vi "Strain - Continuous Input.vi"() -> ()   [LabVIEW 2022 SP3]
doc: "This example demonstrates how to continuously acquire buffered strain measurements using a DAQmx device.\n\nFor instructions on how to connect your signals to the DAQ device, refer to your device documentation."
uses:
  <vilib>/Utility/error.llb/DialogType.ctl
  <vilib>/DAQmx/read.llb/DAQmx Read (Analog 1D Wfm NChan NSamp).vi
  <vilib>/DAQmx/create/channels.llb/DAQmx Create Channel (AI-Strain-Strain Gage).vi
  <vilib>/DAQmx/configure/timing.llb/DAQmx Timing (Sample Clock).vi
  <vilib>/DAQmx/configure/task.llb/DAQmx Configure Logging (TDMS).vi
  <vilib>/DAQmx/configure/trigger.llb/DAQmx Start Trigger (Digital Edge).vi
  <vilib>/DAQmx/configure/trigger.llb/DAQmx Start Trigger (Time).vi
  <vilib>/DAQmx/configure/trigger.llb/DAQmx Start Trigger (Analog Edge).vi
  <vilib>/DAQmx/calibration/calibrationInfo.llb/DAQmx Perform Shunt Calibration Ex (Strain).vi
  <vilib>/DAQmx/miscellaneous.llb/DAQmx Fill In Error Info.vi
  <resource>/objmgr/daqmx.rc
panel:
  in  "Trigger Type":T1(tab)
  in  "Digital Start Trigger Edge":i32(ring)=10280 caption="Edge" items=["Rising"=10280, "Falling"=10171]
  in  "Digital Start Trigger Source":tag="/Dev1/PFI0" caption="Source"
  in  "Digital Pause Trigger Pause When":i32(ring)=10192 caption="Pause When" items=["High"=10192, "Low"=10214]
  in  "Digital Pause Trigger Source":tag="/Dev1/PFI0" caption="Source"
  in  "Analog Start Trigger Level":dbl caption="Level" format="%0.2f"
  in  "Analog Start Trigger Hysteresis":dbl caption="Hysteresis" format="%.2f"
  in  "Analog Start Trigger Slope":i32(ring)=10280 caption="Slope" items=["Rising"=10280, "Falling"=10171]
  in  "Analog Start Trigger Source":string="APFI0" caption="Source"
  in  "Analog Pause Trigger Source":string="APFI0" caption="Source"
  in  "Analog Pause Trigger Pause When":i32(ring)=10093 caption="Pause When" items=["Above Level"=10093, "Below Level"=10107]
  in  "Analog Pause Trigger Level":dbl caption="Level" format="%.2f"
  in  "When":timestamp
  in  "Select Time\nManually":bool
  in  "Strain Gage Information":T2={"Gage Factor"=2.0, "Nominal Gage Resistance"=350.0, "Poisson Ratio"=0.3} {"Nominal Gage Resistance" format="%0.2f"; "Poisson Ratio" format="%0.2f"; "Gage Factor" format="%0.2f"}
  in  "Bridge Information":T3={"Strain Configuration"=10183, "Lead Wire Resistance"=0.0, "Initial Bridge Voltage"=0.0, "Voltage Excitation Source"=10200, "Voltage Excitation Value"=2.5} {"Initial Bridge Voltage" format="%0.2f"; "Voltage Excitation Source" items=["Internal"=10200, "External"=10167, "None"=10230]; "Voltage Excitation Value" format="%0.2f"; "Lead Wire Resistance" format="%0.2f"; "Strain Configuration" items=["Full Bridge I"=10183, "Full Bridge II"=10184, "Full Bridge III"=10185, "Half Bridge I"=10188, "Half Bridge II"=10189, "Quarter Bridge I"=10271, "Quarter Bridge II"=10272]}
  in  "TDMS File Path":path
  in  "Logging Mode":i32(ring)=10231 items=["Off"=10231, "Log and Read"=15842]
  in  "Sample Clock Source":tag="OnboardClock"
  in  "Do Shunt Cal?":bool caption="Enable Shunt Cal"
  in  "Shunt Element Location":i32(ring)=12465 caption="shunt element location" items=["R1"=12465, "R2"=12466, "R3"=12467, "R4"=14813, "None"=10230]
  in  "Shunt Resistance":dbl=100000.0 format="%#.3p"
  in  "Do Offset Null?":bool caption="Enable Offset Null"
  in  "Minimum Value":dbl=-0.001
  in  "Maximum Value":dbl=0.001
  in  "Physical Channel":tag="Dev1/ai0"
  in  "Stop":bool
  out "Waveform Chart":waveform(dbl)[](graph)
  in  "Samples per Loop":i32=100
  in  "Sample Rate":dbl=1000.0
  out "Actual Sample Rate":dbl format="%0.2f"
  # "Channel Settings"
  # "Acquired Data"
  # "Trigger Settings"
  # "Shunt Calibration \nand Offset Null Settings"
  # "Timing Settings"
  # "Logging Settings"
  # "To enable triggers, select a tab above, and configure the settings.\n\nNot all hardware supports all trigger types. Refer to your device documentation for more information."
  # "This trigger type is not supported in continuous sample timing. \n\nRefer to your device documentation for more information on which triggers are supported."
  # "This trigger type is not supported in continuous sample timing. \n\nRefer to your device documentation for more information on which triggers are supported."
  # "If time is not manually set, task will begin after 10 seconds"
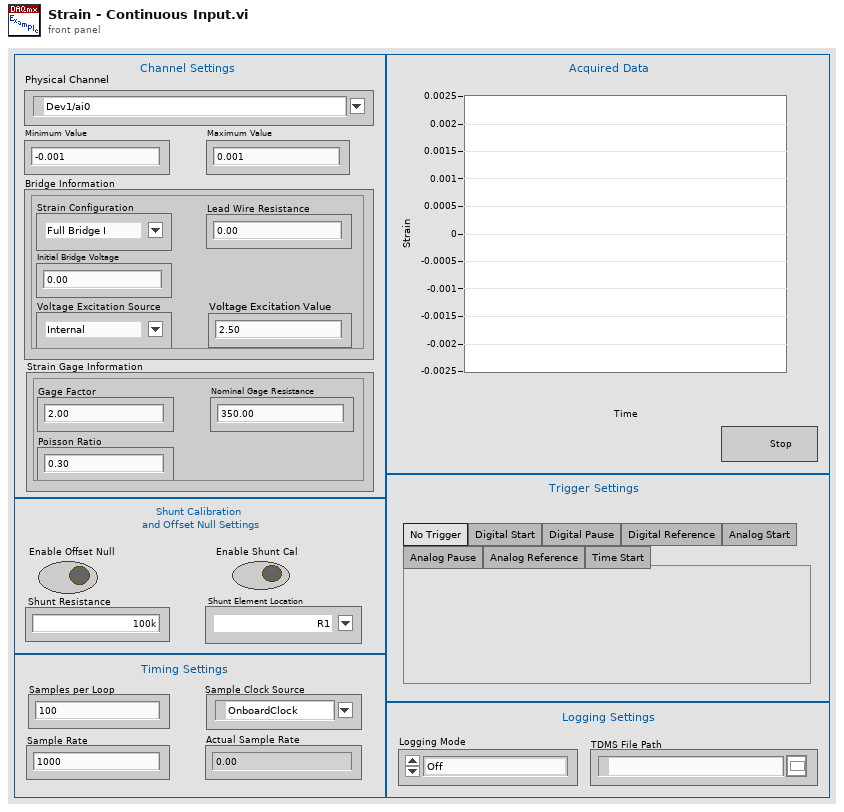
[diagram p1: front panel]
types:
  T1 = enum32{"No Trigger", "Digital Start", "Digital Pause", "Digital Reference", "Analog Start", "Analog Pause", "Analog Reference", "Time Start"}
  T2 = cluster{"Gage Factor":dbl, "Nominal Gage Resistance":dbl, "Poisson Ratio":dbl}
  T3 = cluster{"Strain Configuration":i32, "Lead Wire Resistance":dbl, "Initial Bridge Voltage":dbl, "Voltage Excitation Source":i32, "Voltage Excitation Value":dbl}
  T4 = typedef "DialogType.ctl" = u16
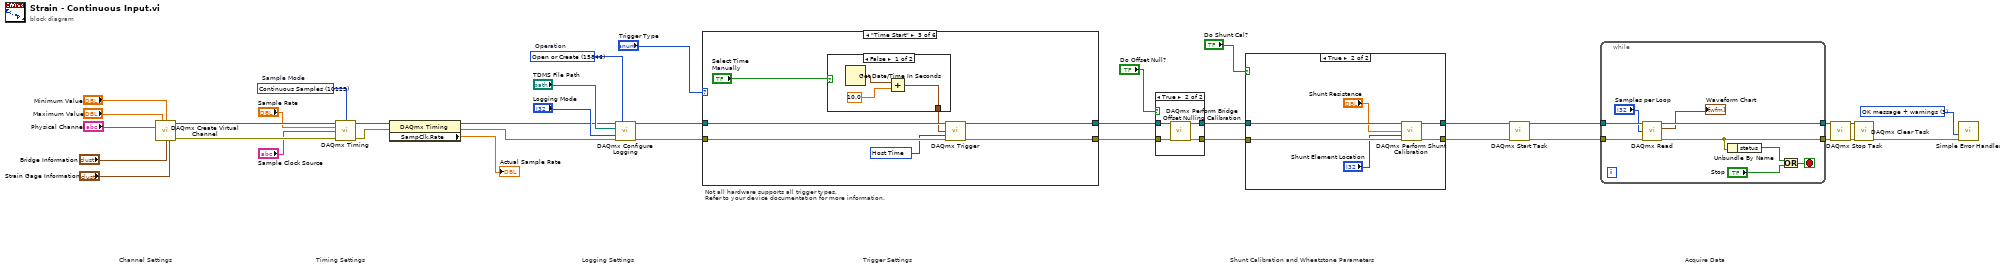
[diagram p0: block diagram]
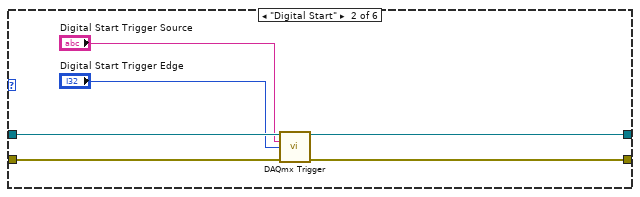
[diagram p3: hidden frame]
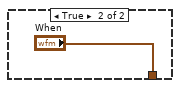
[diagram p4: hidden frame]
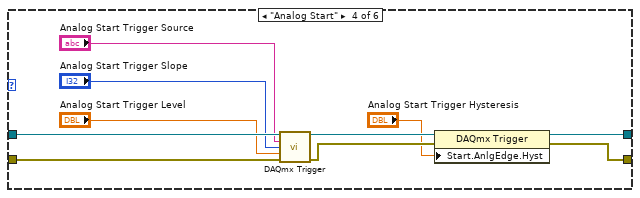
[diagram p5: hidden frame]
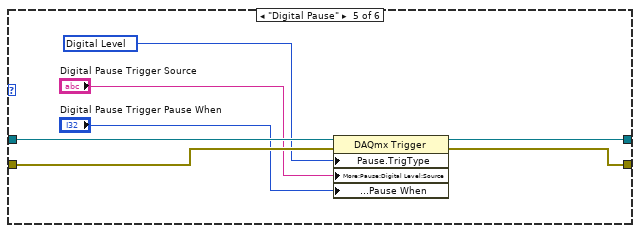
[diagram p6: hidden frame]
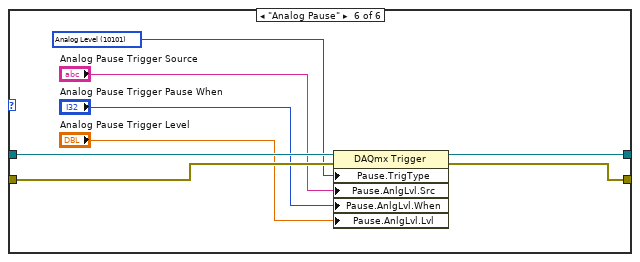
[diagram p7: hidden frame]
diagram:
  w6 = T4 3 items=["no dialog", "OK message", "continue or stop message", "OK message + warnings", "continue/stop + warnings"] ("type of dialog (OK msg:1)")
  w15 = 15846 items=["Open"=10437, "Open or Create"=15846, "Create or Replace"=15847, "Create"=15848]  # Operation
  w35 = 10123 items=["Finite Samples"=10178, "Continuous Samples"=10123, "Hardware Timed Single Point"=12522]  # Sample Mode
  # "Trigger Settings"
  # "Not all hardware supports all trigger types.\nRefer to your device documentation for more information."
  # "Logging Settings"
  # "Acquire Data"
  # "Shunt Calibration and Wheatstone Parameters"
  # "Timing Settings"
  # "Channel Settings"
  n1 = call-poly <vilib>:"DAQmx Create Virtual Channel.vi"("maximum value"="Maximum Value", "minimum value"="Minimum Value", "physical channels"="Physical Channel", "bridge information"="Bridge Information", "strain gage information"="Strain Gage Information") -> ("task out"=w33:refnum<k21>, "error out"=w34:errorcluster)  [unwired: 9 in]
  n2 = call-poly <vilib>:"DAQmx Timing.vi"("task/channels in"=w33, "sample mode"=w35, "rate"="Sample Rate", "source"="Sample Clock Source", "error in"=w34) -> ("task out"=w37:refnum<k21>, "error out"=w36:errorcluster)  [unwired: 9 in]
  n3 = property class="DAQmx Timing"(reference=w37, error in=w36) -> (reference out=w14:refnum<k21>, error out=w13:errorcluster, "SampClk.Rate"=→"Actual Sample Rate":dbl)
  n4 = call-poly <vilib>:"DAQmx Configure Logging.vi"("task/channels in"=w14, "operation"=w15, "file path"="TDMS File Path", "logging mode"="Logging Mode", "error in"=w13) -> ("task out"=w3:refnum<k21>, "error out"=w4:errorcluster)  [unwired: 9 in]
  n5 = case shown="\"Time Start\"" "Trigger Type" {
    tunnel: w3 -> [w39 w45 w52 w66 w73 w81]
    tunnel: w4 -> [w38 w44 w51 w65 w70 w78]
    tunnel: [w39 w43 w50 w63 w72 w80] -> w2
    tunnel: [w38 w42 w49 w62 w71 w79] -> w1
    frame "No Trigger", Default {
    }
    frame "Digital Start" {
      n6 = call-poly <vilib>:"DAQmx Trigger.vi"("task/channels in"=w45, "source"="Digital Start Trigger Source", "edge"="Digital Start Trigger Edge", "error in"=w44) -> ("task out"=w43:refnum<k21>, "error out"=w42:errorcluster)  [unwired: 10 in]
    }
    frame "Time Start" {
      w48 = 16126 items=["Host Time"=16126, "I/O Device Time"=16127] ("timescale")
      n7 = case shown="False" "Select Time\nManually" {
        tunnel: [w54 "When"] -> w46
        frame False {
          n8 = Get Date/Time In Seconds() -> (seconds since 1Jan1904=w55:timestamp)
          n9 = Add(x=w55, y=10.0) -> (x+y=w54:timestamp)
        }
        frame True {
        }
      }
      n10 = call-poly <vilib>:"DAQmx Trigger.vi"("task/channels in"=w52, "when"=w46, "timescale"=w48, "error in"=w51) -> ("task out"=w50:refnum<k21>, "error out"=w49:errorcluster)  [unwired: 10 in]
    }
    frame "Analog Start" {
      n11 = call-poly <vilib>:"DAQmx Trigger.vi"("task/channels in"=w66, "source"="Analog Start Trigger Source", "slope"="Analog Start Trigger Slope", "level"="Analog Start Trigger Level", "error in"=w65) -> ("task out"=w61:refnum<k21>, "error out"=w60:errorcluster)  [unwired: 9 in]
      n12 = property class="DAQmx Trigger"(reference=w61, error in=w60, "Start.AnlgEdge.Hyst"="Analog Start Trigger Hysteresis") -> (reference out=w63:refnum<k21>, error out=w62:errorcluster)
    }
    frame "Digital Pause" {
      w69 = 10152 items=["Analog Level"=10101, "Analog Window"=10103, "Digital Level"=10152, "Digital Pattern"=10398, "None"=10230] ("Pause.TrigType")
      n13 = property class="DAQmx Trigger"(reference=w73, error in=w70, "Pause.TrigType"=w69, "More:Pause:Digital Level:Source"="Digital Pause Trigger Source", "More:Pause:Digital Level:Pause When"="Digital Pause Trigger Pause When") -> (reference out=w72:refnum<k21>, error out=w71:errorcluster)
    }
    frame "Analog Pause" {
      w77 = 10101 items=["Analog Level"=10101, "Analog Window"=10103, "Digital Level"=10152, "Digital Pattern"=10398, "None"=10230] ("Pause.TrigType")
      n14 = property class="DAQmx Trigger"(reference=w81, error in=w78, "Pause.TrigType"=w77, "Pause.AnlgLvl.Src"="Analog Pause Trigger Source", "Pause.AnlgLvl.When"="Analog Pause Trigger Pause When", "Pause.AnlgLvl.Lvl"="Analog Pause Trigger Level") -> (reference out=w80:refnum<k21>, error out=w79:errorcluster)
    }
  }
  n15 = case shown="True" "Do Offset Null?" {
    tunnel: [w83 w87] -> w23
    tunnel: [w82 w86] -> w22
    tunnel: w2 -> [w83 w85]
    tunnel: w1 -> [w82 w84]
    frame False {
    }
    frame True {
      n16 = call <vilib>:"DAQmx Perform Bridge Offset Nulling Calibration.vi"("task/channels in"=w85, "error in"=w84) -> ("task out"=w87:refnum<k21>, "error out"=w86:errorcluster)  [unwired: 12 in]
    }
  }
  n17 = case shown="True" "Do Shunt Cal?" {
    tunnel: w23 -> [w89 w95]
    tunnel: w22 -> [w88 w94]
    tunnel: [w88 w93] -> w18
    tunnel: [w89 w92] -> w19
    frame False {
    }
    frame True {
      n18 = call-poly <vilib>:"DAQmx Perform Shunt Calibration.vi"("task/channels in"=w95, "shunt resistance"="Shunt Resistance", "shunt element location"="Shunt Element Location", "error in"=w94) -> ("task out"=w92:refnum<k21>, "error out"=w93:errorcluster)  [unwired: 10 in]
    }
  }
  n19 = call <vilib>:"DAQmx Start Task.vi"("task/channels in"=w19, "error in"=w18) -> ("task out"=w32:refnum<k21>, "error out"=w31:errorcluster)  [unwired: 12 in]
  n20 = while {
    tunnel: w32 -> [w104]
    tunnel: w31 -> [w103]
    tunnel: [w100] -> w8
    tunnel: [w101] -> w9
    stop <- w102 stop-if-true
    n21 = call-poly <vilib>:"DAQmx Read.vi"("task/channels in"=w104, "number of samples per channel"="Samples per Loop", "error in"=w103) -> ("task out"=w101:refnum<k21>, "data"=→"Waveform Chart":waveform(dbl)[], "error out"=w100:errorcluster)  [unwired: 10 in]
    n22 = Unbundle By Name(w100) -> ("status"=w99:bool)
    n23 = Or(x=w99, y="Stop") -> (x .or. y?=w102:bool)
  }
  n24 = call <vilib>:"DAQmx Stop Task.vi"("task/channels in"=w9, "error in"=w8) -> ("task out"=w10:refnum<k21>, "error out"=w7:errorcluster)  [unwired: 12 in]
  n25 = call <vilib>:"DAQmx Clear Task.vi"("task in"=w10, "error in"=w7) -> ("error out"=w30:errorcluster)  [unwired: 13 in]
  n26 = call <vilib>:"Simple Error Handler.vi"("type of dialog (OK msg:1)"=w6, "error in (no error)"=w30) -> ()  [unwired: 3 in, 5 out]
